vi "Set Assert VI UID.vi"(8 "error in (no error)":errorcluster, 10 "GObj Refnum":refnum<vi>, 11 "Assert VI Path":path) -> (0 "error out":errorcluster)   [LabVIEW 2016]
doc: "Identifies the referenced nodes UID and sets the UID constant to that value"
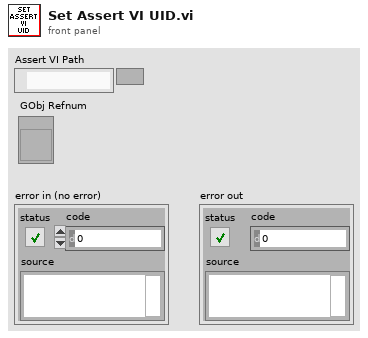
[diagram p1: front panel]
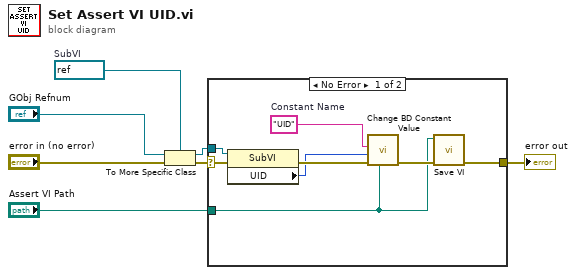
[diagram p0: block diagram]
diagram:
  w5 = refnum<vi> refnum  # SubVI
  n1 = To More Specific Class(target class=w5, reference="GObj Refnum", error in="error in (no error)") -> (specific class reference=w3:refnum<vi>, error out=w4:errorcluster)
  n2 = case shown="No Error" w4 {
    selector: w4 -> [w14 w16]
    tunnel: w3 -> [w15 _]
    tunnel: "Assert VI Path" -> [w8 _]
    tunnel: [w9 w16] -> w1
    frame No Error {
      w11 = "UID"  # Constant Name
      n3 = property class="SubVI"(reference=w15, error in=w14) -> (error out=w13:errorcluster, "UID"=w12:i32)  [unwired: 1 out]
      n4 = call "Change BD Constant Value.vi"("Assert VI Path"=w8, "error in (no error)"=w13, "Data Value"=w12, "Constant Name"=w11) -> ("error out"=w10:errorcluster)  [unwired: 7 in]
      n5 = call "Save VI.vi"("error in (no error)"=w10, "Assert VI Path"=w8) -> ("error out"=w9:errorcluster)  [unwired: 9 in]
    }
    frame Error {
    }
  }
  "error out" <- w1
